vi "ExSubCreateFileDisplayQU16.vi"(2 "error in (no error)":errorcluster, 3 "File and Display Name":string, 4 "Pulser Handle":u32, 5 "Camera Handle":u32) -> (0 "error out":errorcluster, 1 "Handles Out":T1)   [LabVIEW 2012]
panel:
  # "ExSubCreateFileDisplay:\nThis is a SubVI that creates a file, display and image \nobjects and returns the handles bundled in a cluster \nthat includes a pulser and camera handle"
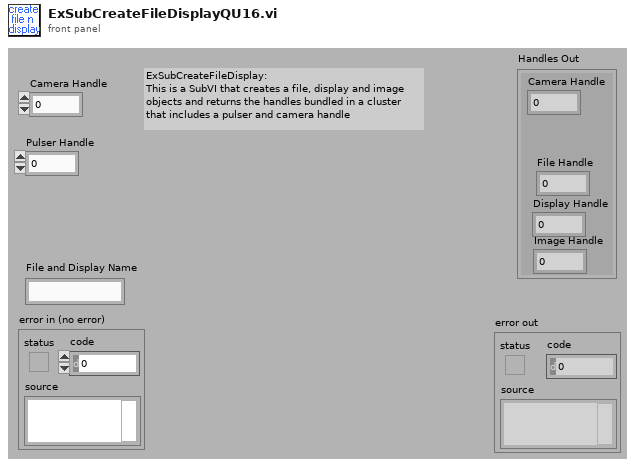
[diagram p1: front panel]
types:
  T1 = cluster{"Camera Handle":u32, "File Handle":u32, "Display Handle":u32, "Image Handle":u32}
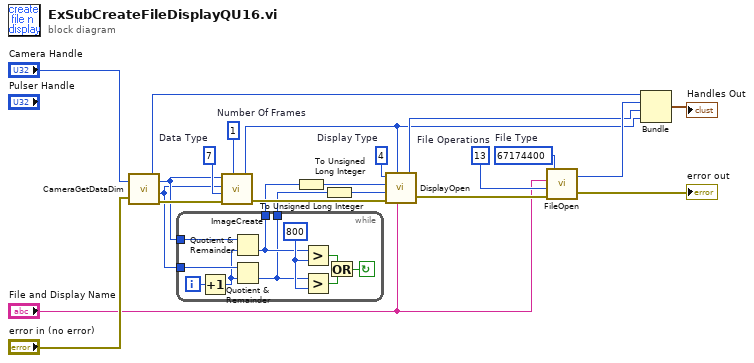
[diagram p0: block diagram]
diagram:
  w11 = u32 1  # Number Of Frames
  w12 = u32 4  # Display Type
  w13 = u32 7  # Data Type
  w15 = 13  # File Operations
  w16 = 67174400  # File Type
  n1 = call <userlib>:"CameraGetDataDim.vi"("Camera Handle"="Camera Handle", "error in"="error in (no error)") -> ("Camera Handle"=w17:u32, "Xdim"=w10:u32, "Ydim"=w9:u32, "error out"=w23:errorcluster)
  n2 = while {
    tunnel: w10 -> [w32]
    tunnel: w9 -> [w31]
    tunnel: [w26] -> w8
    tunnel: [w25] -> w7
    i -> [w30]
    stop <- w27 continue-if-true
    w33 = 800
    n3 = Increment(x=w30) -> (x+1=w24:i32)
    n4 = Quotient & Remainder(x=w32, y=w24) -> (floor(x/y)=w26:u32)  [unwired: 1 out]
    n5 = Quotient & Remainder(x=w31, y=w24) -> (floor(x/y)=w25:u32)  [unwired: 1 out]
    n6 = Greater?(x=w26, y=w33) -> (0:w29:bool)
    n7 = Greater?(x=w25, y=w33) -> (0:w28:bool)
    n8 = Or(x=w29, y=w28) -> (x .or. y?=w27:bool)
  }
  n9 = call <userlib>:"ImageCreate.vi"("X dimension"=w10, "Y dimension"=w9, "Data Type"=w13, "error in"=w23, "Number Of Frames"=w11) -> ("Image Handle"=w2:u32, "error out"=w22:errorcluster)
  n10 = To Unsigned Long Integer(number=w8) -> (unsigned 32bit integer=w6:u32)
  n11 = To Unsigned Long Integer(number=w7) -> (unsigned 32bit integer=w5:u32)
  n12 = call <userlib>:"DisplayOpen.vi"("Display Title"="File and Display Name", "Image Handle"=w2, "error in"=w22, "Display Height"=w5, "Display Width"=w6, "Display Type"=w12) -> ("error out"=w21:errorcluster, "Display Handle"=w3:u32)
  n13 = call <userlib>:"FileOpen.vi"("error in"=w21, "File Operations"=w15, "FileName"="File and Display Name", "File Type"=w16) -> ("error out"=→"error out":errorcluster, "File Handle"=w4:u32)
  n14 = Bundle("Camera Handle"=w17, "File Handle"=w4, "Display Handle"=w3, "Image Handle"=w2) -> (→"Handles Out":T1)  [unwired: 1 in]
